vi "start.vi"(8 "error in (no error)":errorcluster, 11 "Counter in":refnum<class "Counter.lvclass">) -> (0 "error out":errorcluster, 3 "Counter out":refnum<class "Counter.lvclass">)   [LabVIEW 2013, in "Counter.lvclass"]
uses:
  Counter.lvclass
  Counter.lvclass/Counter.ctl
  Globals.vi
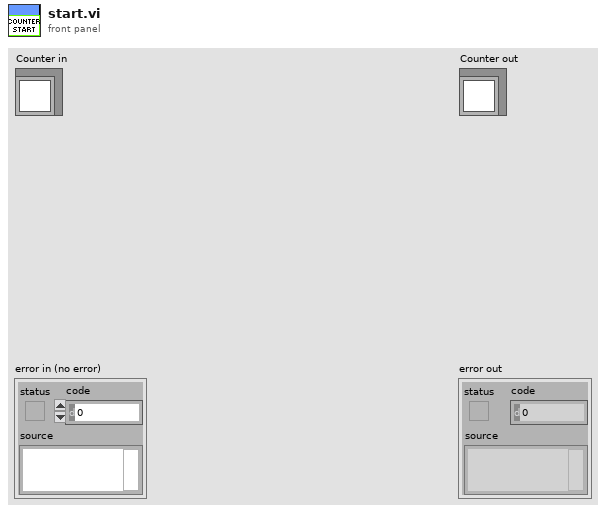
[diagram p1: front panel]
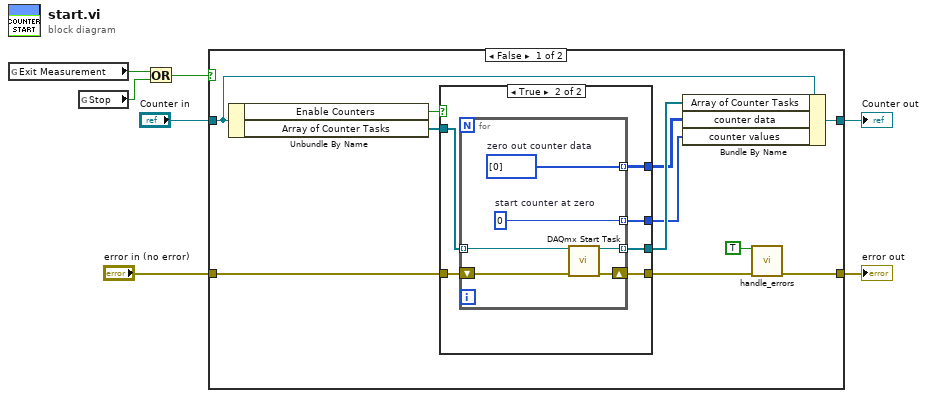
[diagram p0: block diagram]
diagram:
  n1 = global read "Globals.vi" "Exit Measurement"() -> (w3:bool)
  n2 = global read "Globals.vi" "Stop"() -> (w4:bool)
  n3 = Or(x=w3, y=w4) -> (x .or. y?=w2:bool)
  n4 = case shown="False" w2 {
    tunnel: [w9 w33] -> w5
    tunnel: [w15 w34] -> w6
    tunnel: "Counter in" -> [w16 w34]
    tunnel: "error in (no error)" -> [w8 w33]
    frame False {
      n5 = Unbundle By Name(w16) -> ("Enable Counters"=w18:bool, "Array of Counter Tasks"=w17:refnum<k21>[])
      n6 = case shown="True" w18 {
        tunnel: w17 -> [w20 w26]
        tunnel: [w19 w25] -> w11
        tunnel: [w20 w24] -> w14
        tunnel: [_ w23] -> w12
        tunnel: [_ w22] -> w13
        tunnel: w8 -> [w19 w21]
        frame False {
        }
        frame True {
          n7 = for {
            tunnel: w26 -> [w32] mode=indexing
            shift-right: [w30] -> w25
            shift-left: w21 -> [w31]
            tunnel: [w29] -> w24 mode=indexing
            tunnel: [w28] -> w23 mode=indexing
            tunnel: [w27] -> w22 mode=indexing
            w27 = u32[] [0]  # zero out counter data
            w28 = u32 0  # start counter at zero
            n8 = call <vilib>:"DAQmx Start Task.vi"("task/channels in"=w32, "error in"=w31) -> ("task out"=w29:refnum<k21>, "error out"=w30:errorcluster)  [unwired: 12 in]
          }
        }
      }
      n9 = Bundle By Name(cluster=w16, "Array of Counter Tasks"=w14, "counter data"=w13, "counter values"=w12) -> (w15:refnum<class "Counter.lvclass">)
      n10 = call "handle_errors.vi"("Exit Operation"=TRUE ("Exit Measurement"), "error in (no error)"=w11) -> ("error out"=w9:errorcluster)  [unwired: 13 in]
    }
    frame True {
    }
  }
  "error out" <- w5
  "Counter out" <- w6
